vi "Scope.vi"(7 "JPG":refnum<vi>, 10 "queueName":string="PV_script", 11 "Console Reference":refnum<vi>) -> ()   [LabVIEW 2022 SP3]
uses:
  <vilib>/Utility/file.llb/Write Delimited Spreadsheet (DBL).vi
panel:
  in  "Ctrl C":bool
  in  "start":bool
  in  "Save":bool
  in  "python":string
  in  "Send":bool
  in  "Clear":bool
  in  "Tab Control":enum32{"Chart", "Scope", "XY Plot", "Gauges"}(tab)
  out "Chart":dbl[][](graph)
  out "Graph":dbl[](graph)
  out "XY Plot":cluster{dbl[], dbl[]}[](graph)
  out "Gauge":dbl[](array[knob]) scale=-100.0..100.0
  out "Last Line":string
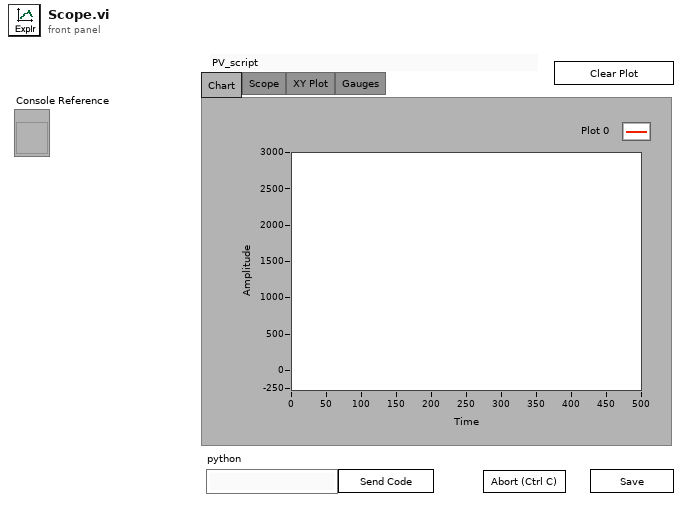
[diagram p1: front panel]
types:
  T1 = enum16{"Not data", "single values", "XY pairs", "Arrays"}
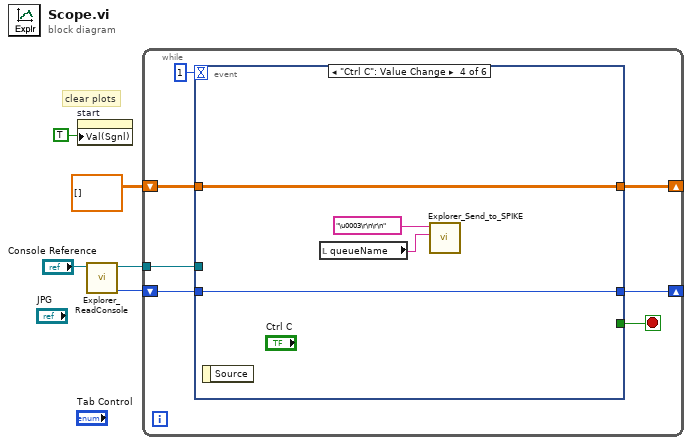
[diagram p0: block diagram]
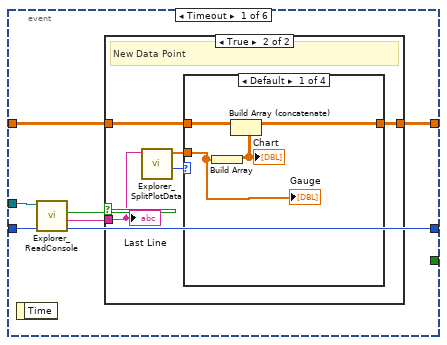
[diagram p2: hidden frame]
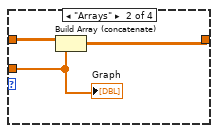
[diagram p4: hidden frame]
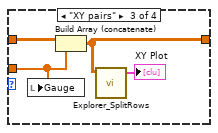
[diagram p5: hidden frame]
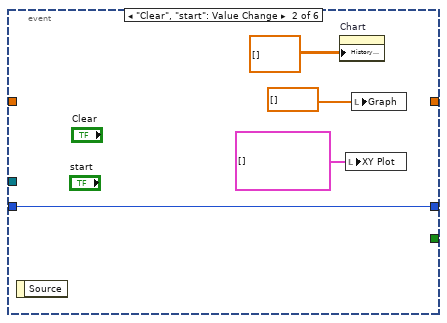
[diagram p7: hidden frame]
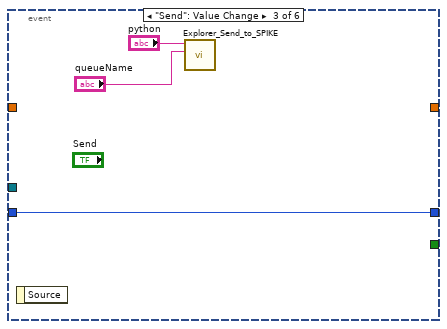
[diagram p8: hidden frame]
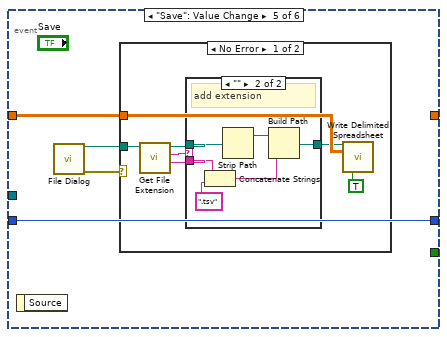
[diagram p9: hidden frame]
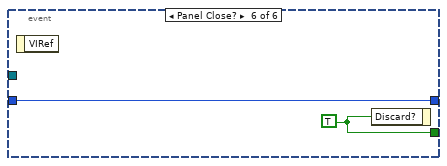
[diagram p12: hidden frame]
diagram:
  # "clear plots"
  n1 = property on="start" class="Bool (strict)"("Val(Sgnl)"=TRUE ("Value (Signaling)")) -> ()  [unwired: 2 in, 2 out]
  n2 = call "Explorer_ReadConsole.vi"("String in"="Console Reference") -> ("index out"=w4:i32, "String out"=w3:refnum<vi>)  [unwired: 6 in, 3 out]
  n3 = while {
    shift-right: [w10] -> _
    shift-left: w4 -> [w9]
    shift-right: [w6] -> _
    shift-left: dbl[][] [] -> [w8]
    tunnel: w3 -> [w7]
    stop <- w11 stop-if-true
    n4 = event shown="[3] \"Ctrl C\": Value Change" {
      selector: _ -> [_ _ _ _ _ _]
      dyn-events: _ -> [_ _ _ _ _ _]
      timeout: 1 -> [_ _ _ _ _ _]
      tunnel: [_ _ _ _ _ w68] -> w11
      tunnel: [w16 w41 w44 w47 w52 w67] -> w10
      tunnel: w9 -> [w17 w41 w44 w47 w52 w67]
      tunnel: w8 -> [w19 _ _ w48 w51 _]
      tunnel: [w18 _ _ w48 _ _] -> w6
      tunnel: w7 -> [w13 _ _ _ _ _]
      event Timeout {
        n5 = event-data() -> ()  [unwired: 1 in, 1 out]
        n6 = call "Explorer_ReadConsole.vi"("index in"=w17, "String in"=w13) -> ("index out"=w16:i32, "New Line"=w15:string, "New point?"=w14:bool)  [unwired: 5 in, 2 out]
        n7 = case shown="True" w14 {
          tunnel: w15 -> [_ w25]
          tunnel: w19 -> [w20 w24]
          tunnel: [w20 w23] -> w18
          frame False {
            # "nothing new"
          }
          frame True {
            # "New Data Point"
            n8 = call "Explorer_SplitPlotData.vi"("Value"=w25) -> ("Data type"=w22:T1, "Array"=w21:dbl[])  [unwired: 9 in]
            n9 = case shown="Default" w22 {
              tunnel: w24 -> [w29 w32 w36 w37]
              tunnel: [w28 w30 w33 w37] -> w23
              tunnel: w21 -> [w27 w31 w34 _]
              frame Default {
                n10 = Build Array(w27) -> (w26:dbl[][])
                "Chart" <- w26
                n11 = Build Array (concatenate)(w29, w26) -> (w28:dbl[][])
                "Gauge" <- w27
              }
              frame "Arrays" {
                n12 = Build Array (concatenate)(w32, w31) -> (w30:dbl[][])
                "Graph" <- w31
              }
              frame "XY pairs" {
                n13 = local write "Gauge"(w34) -> ()
                n14 = Build Array (concatenate)(w36, w34) -> (w33:dbl[][])
                n15 = call "Explorer_SplitRows.vi"("Array in"=w33) -> ("XY Plot"=→"XY Plot":cluster{dbl[], dbl[]}[])  [unwired: 10 in]
              }
              frame "Not data" {
              }
            }
            "Last Line" <- w25
          }
        }
      }
      event "Clear", "start": Value Change {
        n16 = event-data() -> ()  [unwired: 1 in, 1 out]
        n17 = property on="Chart" class="WFChart (strict)"("History Data"=dbl[][] []) -> ()  [unwired: 2 in, 2 out]
        n18 = local write "XY Plot"(cluster{dbl[], dbl[]}[] [] ("XY Plot")) -> ()
        n19 = local write "Graph"(dbl[] []) -> ()
      }
      event "Send": Value Change {
        n20 = event-data() -> ()  [unwired: 1 in, 1 out]
        n21 = call "Explorer_Send_to_SPIKE.vi"("queueName"="queueName", "python"="python") -> ()  [unwired: 9 in, 1 out]
      }
      event "Ctrl C": Value Change {
        n22 = event-data() -> ()  [unwired: 1 in, 1 out]
        n23 = local read "queueName"() -> (w45:string)
        n24 = call "Explorer_Send_to_SPIKE.vi"("queueName"=w45, "python"="\u0003\r\n\r\n" ("function name")) -> ()  [unwired: 9 in, 1 out]
      }
      event "Save": Value Change {
        n25 = event-data() -> ()  [unwired: 1 in, 1 out]
        n26 = call "File Dialog"() -> ("selected path"=w50:path, "error out"=w49:errorcluster)  [unwired: 12 in, 2 out]
        n27 = case shown="No Error" w49 {
          tunnel: w51 -> [w59 _]
          tunnel: w50 -> [w57 _]
          frame No Error {
            n28 = call <vilib>:"Get File Extension.vi"("file"=w57) -> ("filename without extension"=w53:string, "lowercase file extension"=w56:string, "dup file"=w54:path)  [unwired: 6 in, 2 out]
            n29 = case shown="\"\"" w56 {
              tunnel: [w60 w62] -> w55
              tunnel: w54 -> [w60 w64]
              tunnel: w53 -> [_ w66]
              frame Default {
              }
              frame "" {
                # "add extension"
                n30 = Concatenate Strings(w66, ".tsv" ("pattern (all files)")) -> (w61:string)
                n31 = Strip Path(path=w64) -> (stripped path=w63:path)  [unwired: 1 out]
                n32 = Build Path(base path=w63, name or relative path=w61) -> (appended path=w62:path)
              }
            }
            n33 = call-poly <vilib>:"Write Delimited Spreadsheet.vi"("file path (dialog if empty)"=w55, "2D data"=w59, "transpose? (no:F)"=TRUE) -> ()  [unwired: 11 in, 2 out]
          }
          frame Error {
          }
        }
      }
      event Panel Close? {
        w68 = TRUE ("Discard?")
        n34 = event-data() -> ()  [unwired: 1 in, 1 out]
        n35 = event-data("Discard?"=w68) -> ()  [unwired: 1 in, 1 out]
      }
    }
  }
